vi "DC MOTOR CONTROLL.vi"() -> ()   [LabVIEW 2017]
uses:
  <vilib>/LabVIEW Interface for Arduino/Type Defs/Board Type.ctl
  <vilib>/LabVIEW Interface for Arduino/Type Defs/Connection Type.ctl
  <vilib>/LabVIEW Interface for Arduino/LabVIEW Interface for Arduino.lvlib
panel:
  in  "MODE SELECTION":enum32{" FORWARD", "REVERSE"}(radio)
  out "ON/OFF":bool
  in  "stop":bool
  in  "SPEED":dbl(slide) scale=0.0..100.0
  in  "EN":bool
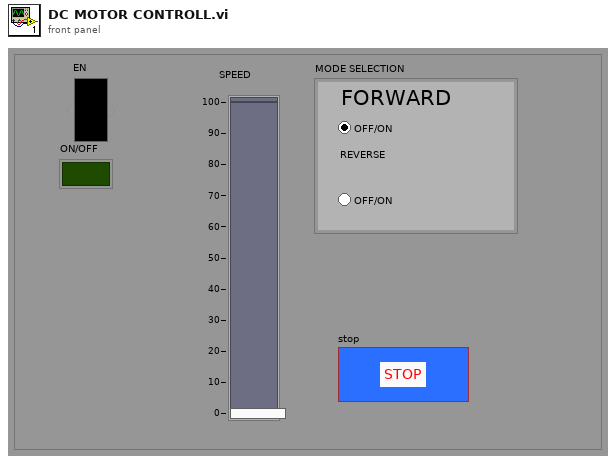
[diagram p1: front panel]
types:
  T1 = typedef "LabVIEW Interface for Arduino.lvlib/Connection Type.ctl" = enum8{"USB / Serial", "XBEE", "BlueSmirf (Bluetooth)"}
  T2 = typedef "LabVIEW Interface for Arduino.lvlib/Board Type.ctl" = enum16{"Uno", "Dimuelanove w/Atmega 328", "Mega 2560"}
  T3 = typedef "LabVIEW Interface for Arduino.lvlib/Arduino Resource.ctl" = cluster{"VISA resource":refnum<visa-resource-name>, "Board Type":T2, "Connection Type":enum8{"USB / Serial"}, "Bytes Per Packet (15)":u8}
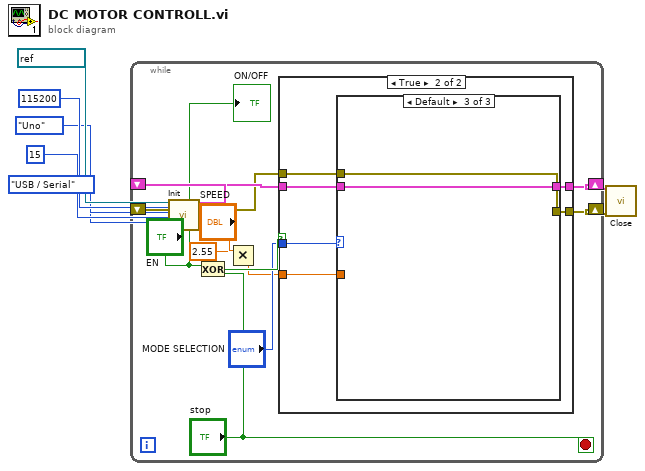
[diagram p0: block diagram]
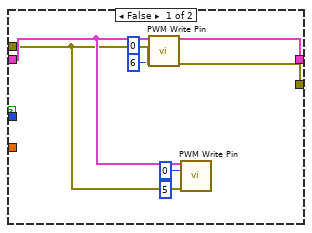
[diagram p2: hidden frame]
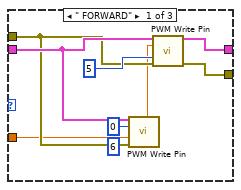
[diagram p3: hidden frame]
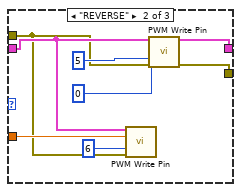
[diagram p4: hidden frame]
diagram:
  n1 = call <vilib>:"Init.vi"("VISA resource"=refnum<visa-resource-name> "COM19", "Baud Rate (115200)"=u32 115200, "Board Type (Uno)"=Board_Type."Uno", "Bytes Per Packet (15)"=u32 15, "Connection Type (USB/Serial)"=Connection_Type."USB / Serial") -> ("Arduino Resource"=w4:T3, "error out"=w3:errorcluster)  [unwired: 13 in]
  n2 = while {
    shift-right: [w18] -> w2
    shift-left: w4 -> [w20]
    shift-right: [w17] -> w1
    shift-left: w3 -> [w19]
    stop <- "stop" stop-if-true
    n3 = Exclusive Or(1:"stop", 2:"EN") -> (0:w16:bool)
    n4 = Multiply(x="SPEED", y=2.55) -> (x*y=w11:dbl)
    n5 = case shown="True" w16 {
      tunnel: w20 -> [w28 w34]
      tunnel: w19 -> [w27 w33]
      tunnel: [w22 w32] -> w18
      tunnel: [w21 w31] -> w17
      tunnel: "MODE SELECTION" -> [_ w30]
      tunnel: w11 -> [_ w29]
      frame False {
        n6 = call <vilib>:"PWM Write Pin.vi"("Arduino Resource"=w28, "Duty Cycle (0 - 255)"=u8 0, "PWM Pin (3)"=u8 6, "error in"=w27) -> ("Arduino Resource"=w22:T3, "error out"=w21:errorcluster)  [unwired: 10 in]
        n7 = call <vilib>:"PWM Write Pin.vi"("Arduino Resource"=w28, "Duty Cycle (0 - 255)"=u8 0, "PWM Pin (3)"=u8 5, "error in"=w27) -> ()  [unwired: 10 in, 2 out]
      }
      frame True {
        n8 = case shown="Default" w30 {
          tunnel: w34 -> [w39 w45 w51]
          tunnel: w33 -> [w38 w44 w52]
          tunnel: [w41 w50 w51] -> w32
          tunnel: [w40 w49 w52] -> w31
          tunnel: w29 -> [w35 w46 _]
          frame " FORWARD" {
            n9 = call <vilib>:"PWM Write Pin.vi"("Arduino Resource"=w39, "Duty Cycle (0 - 255)"=u8 0, "PWM Pin (3)"=u8 6, "error in"=w38) -> ()  [unwired: 10 in, 2 out]
            n10 = call <vilib>:"PWM Write Pin.vi"("Arduino Resource"=w39, "Duty Cycle (0 - 255)"=w35, "PWM Pin (3)"=u8 5, "error in"=w38) -> ("Arduino Resource"=w41:T3, "error out"=w40:errorcluster)  [unwired: 10 in]
          }
          frame "REVERSE" {
            n11 = call <vilib>:"PWM Write Pin.vi"("Arduino Resource"=w45, "Duty Cycle (0 - 255)"=w46, "PWM Pin (3)"=u8 6, "error in"=w44) -> ()  [unwired: 10 in, 2 out]
            n12 = call <vilib>:"PWM Write Pin.vi"("Arduino Resource"=w45, "Duty Cycle (0 - 255)"=u8 0, "PWM Pin (3)"=u8 5, "error in"=w44) -> ("Arduino Resource"=w50:T3, "error out"=w49:errorcluster)  [unwired: 10 in]
          }
          frame Default {
          }
        }
      }
    }
    "ON/OFF" <- "EN"
  }
  n13 = call <vilib>:"Close.vi"("Arduino Resource"=w2, "error in"=w1) -> ()  [unwired: 13 in, 1 out]
